vi "RF FC limits set.vi"(8 "error in (no error)":errorcluster, 10 "detected mmWave adapters":T1[](array[typedef]) {"detected mmWave adapters"."serial number" format="%.0x"}, 11 "reference in":refnum<class "mmWave instrument.lvclass">) -> (0 "error out":errorcluster, 3 "reference out":refnum<class "mmWave instrument.lvclass">)   [LabVIEW 2019, in "mmWave instrument.lvclass"]
doc: "Set RF limits based on operation mode and detected RF heads"
uses:
  mmWave instrument.lvclass
  Low-level/TypeDefs/Detected mmWave Adapters.ctl
  <vilib>/userdefined/High Color/nirio_resource_hc.ctl
  Low-level/TypeDefs/mmWave Adapter Information.ctl
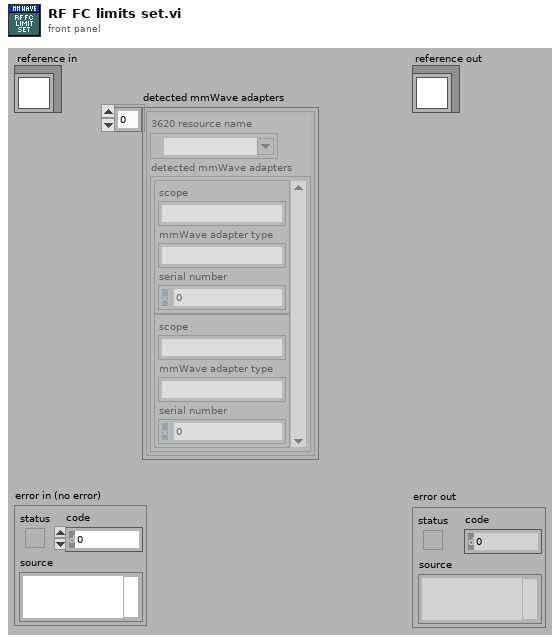
[diagram p1: front panel]
types:
  T1 = typedef "Detected mmWave Adapters.ctl" = cluster{"3620 resource name":T2, "detected mmWave adapters":T3[]}
  T2 = typedef "nirio_resource_hc.ctl" = tag
  T3 = typedef "mmWave Adapter Information.ctl" = cluster{"scope":string, "mmWave adapter type":string, "serial number":u64}
  T4 = typedef "mmWave instrument.lvclass/ObjectAttributesRef.ctl" = refnum<data-value>
  T5 = typedef "mmWave instrument.lvclass/ObjectAttributes.ctl" = cluster{"mode":T6, "instr state":T7, "Max Fs":dbl, "Equalization coeff":cdb[], "LO sync en":bool, "Trig sync en":bool, "LO sources":T8, "LO Export":T9, "Fc.range":cluster{"min":dbl, "max":dbl}, "Sync mode":T10, "equalization en":bool, "sequence":string[]}
  T6 = typedef "mmWave instrument.lvclass/Instrument mode.ctl" = enum16{"RF", "IF", "BB"}
  T7 = typedef "mmWave instrument.lvclass/Instrument state.ctl" = enum16{"Off", "Initialization", "Configuration", "Running", "Calibration"}
  T8 = typedef "mmWave HW Control.lvlib/LO sources.ctl" = cluster{"RX/LO1 src":string, "TX/LO1 src":string, "LO2 src":string}
  T9 = typedef "mmWave HW Control.lvlib/LO export.ctl" = cluster{"TX LO1 export":bool, "TX LO1 export level":dbl, "RX LO1 export":bool, "RX LO1 export level":dbl, "LO2 export":bool, "LO2 export level":dbl}
  T10 = typedef "mmWave instrument.lvclass/Sync mode.ctl" = enum16{"Slave", "Master"}
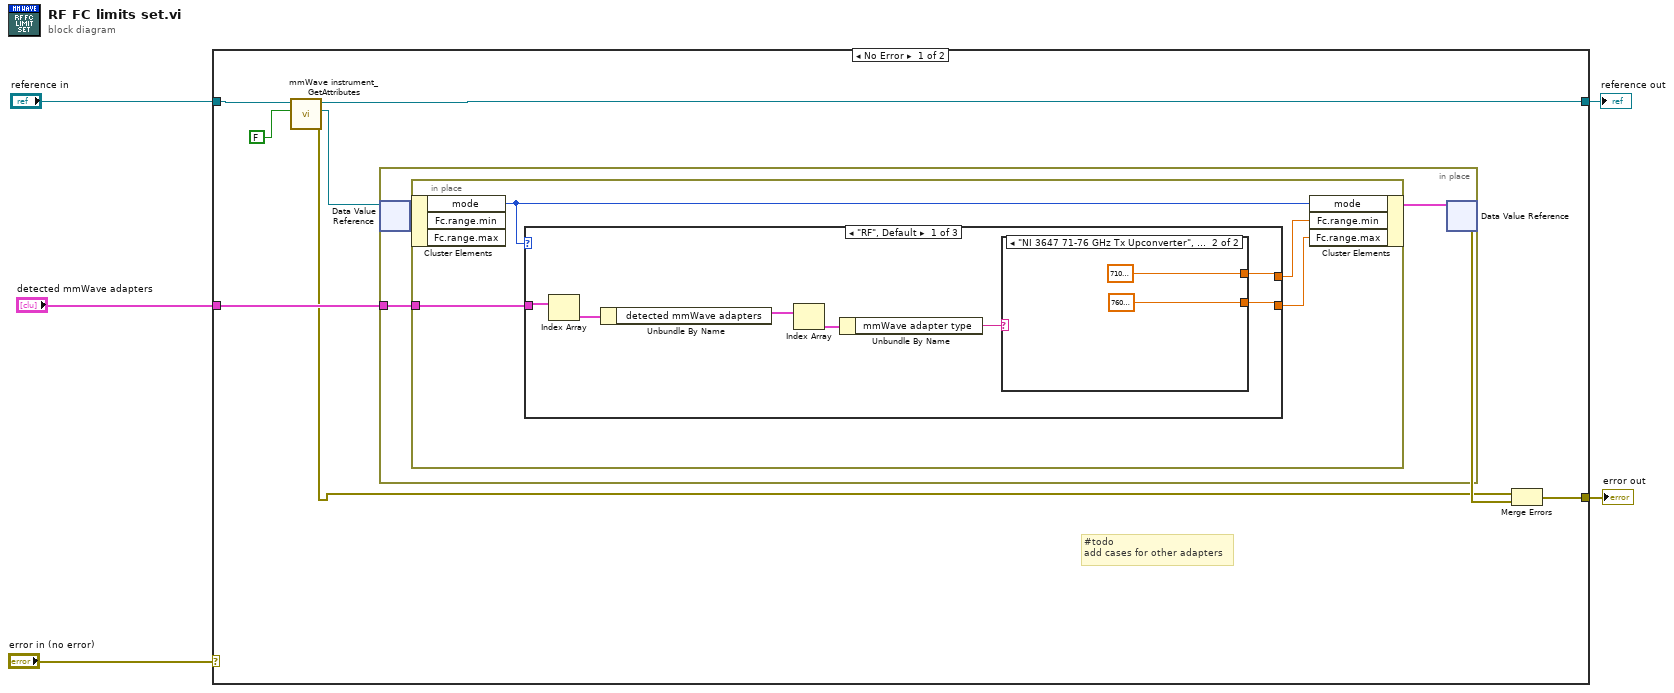
[diagram p0: block diagram]
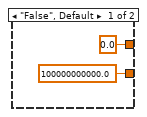
[diagram p2: hidden frame]
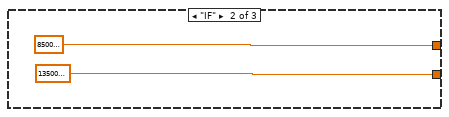
[diagram p3: hidden frame]
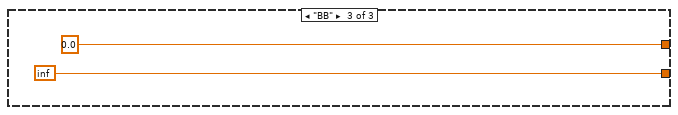
[diagram p4: hidden frame]
diagram:
  n1 = case shown="No Error" "error in (no error)" {
    selector: "error in (no error)" -> [_ w37]
    tunnel: [w6 w37] -> w4
    tunnel: [w13 w36] -> w2
    tunnel: "reference in" -> [w12 w36]
    tunnel: "detected mmWave adapters" -> [w8 _]
    frame No Error {
      # "#todo\nadd cases for other adapters"
      n2 = call "mmWave instrument_GetAttributes.vi"("return data? (T)"=FALSE, "reference in"=w12) -> ("error out"=w7:errorcluster, "attributes ref"=w9:T4, "reference out"=w13:refnum<class "mmWave instrument.lvclass">)  [unwired: 6 in, 1 out]
      n3 = in-place {
        in-place-border: w8 -> [w14]
        n4 = in-place-dvr #1(w9) -> (w15:T5)  [unwired: 1 out]
        n5 = in-place {
          in-place-border: w14 -> [w17]
          n6 = in-place-cluster #2(w15) -> ("mode"=w20:T6)  [unwired: 2 out]
          n7 = case shown="\"RF\", Default" w20 {
            tunnel: [w22 8500000000.0 0.0] -> w19
            tunnel: [w21 13500000000.0 inf] -> w18
            tunnel: w17 -> [w27 _ _]
            frame "RF", Default {
              n8 = Index Array(array=w27) -> (element=w26:T1)  [unwired: 1 in]
              n9 = Unbundle By Name(w26) -> ("detected mmWave adapters"=w25:T3[])
              n10 = Index Array(array=w25) -> (element=w24:T3)  [unwired: 1 in]
              n11 = Unbundle By Name(w24) -> ("mmWave adapter type"=w23:string)
              n12 = case shown="\"NI 3647 71-76 GHz Tx Upconverter\", \"NI 3657 71-76 GHz Rx Downconverter\"" w23 {
                tunnel: [0.0 71000000000.0] -> w22
                tunnel: [100000000000.0 76000000000.0] -> w21
                frame "False", Default {
                }
                frame "NI 3647 71-76 GHz Tx Upconverter", "NI 3657 71-76 GHz Rx Downconverter" {
                }
              }
            }
            frame "IF" {
            }
            frame "BB" {
            }
          }
          n13 = in-place-cluster #2("mode"=w20, "Fc.range.min"=w19, "Fc.range.max"=w18) -> (w16:T5)
        }
        n14 = in-place-dvr #1(w16) -> (w10:errorcluster)  [unwired: 1 out]
      }
      n15 = Merge Errors(w7, w10) -> (w6:errorcluster)
    }
    frame Error {
    }
  }
  "error out" <- w4
  "reference out" <- w2
